vi "Check Histogram Options.vi"(8 "error in (no error)":errorcluster, 11 "Histogram Options in":T1 {"Max Histogram Size" format="%.0e"}) -> (0 "error out":errorcluster, 1 "Cancelled?":bool, 3 "Histogram Options out":T1 {"Max Histogram Size" format="%.0e"})   [LabVIEW 2021, in "Histogram Window.lvlib"]
uses:
  Histogram Window.lvlib
  Linear Histogram Options.ctl
  Histogram Bin Option.ctl
  Histogram Bin Position.ctl
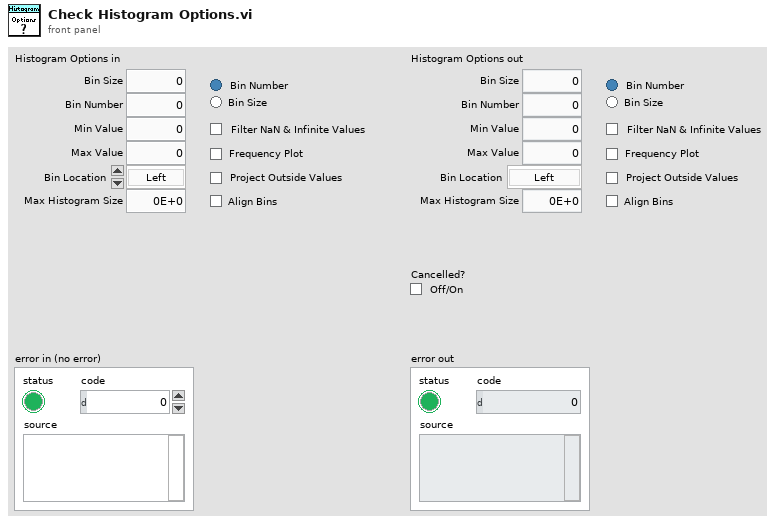
[diagram p1: front panel]
types:
  T1 = typedef "Histogram Window.lvlib/Linear Histogram Options.ctl" = cluster{"Bin Size":dbl, "Bin Number":i32, "Bin Option":T2, "Min Value":dbl, "Max Value":dbl, "Filter NaN & Infinite Values":bool, "Frequency Plot":bool, "Align Bins":bool, "Bin Location":T3, "Project Outside Values":bool, "Max Histogram Size":i32}
  T2 = typedef "Histogram Window.lvlib/Histogram Bin Option.ctl" = enum32{"Bin Number", "Bin Size"}
  T3 = typedef "Histogram Window.lvlib/Histogram Bin Position.ctl" = enum16{"Left", "Center", "Right"}
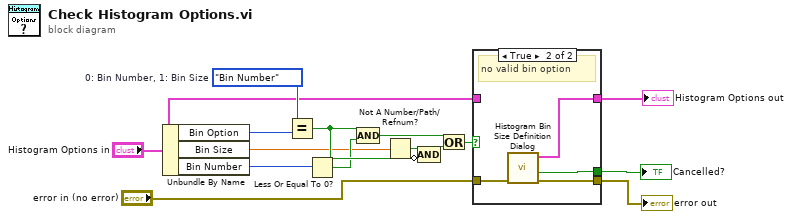
[diagram p0: block diagram]
diagram:
  w9 = Histogram_Bin_Option."Bin Number"  # 0: Bin Number, 1: Bin Size
  n1 = Unbundle By Name("Histogram Options in") -> ("Bin Option"=w8:T2, "Bin Size"=w5:dbl, "Bin Number"=w7:i32)
  n2 = Equal?(x=w9, y=w8) -> (x = y?=w12:bool)
  n3 = Less Or Equal To 0?(x=w7) -> (x <= 0?=w10:bool)
  n4 = Compound Arithmetic op=AND(w12, w10) -> (w13:bool)
  n5 = Not A Number/Path/Refnum?(number/path/refnum=w5) -> (NaN/Path/Refnum?=w11:bool)
  n6 = Compound Arithmetic op=AND(w11, invert w12) -> (w14:bool)
  n7 = Or(x=w13, y=w14) -> (x .or. y?=w15:bool)
  n8 = case shown="True" w15 {
    tunnel: [_ w19] -> w2
    tunnel: [w17 w21] -> w3
    tunnel: "error in (no error)" -> [w17 w20]
    tunnel: [w16 w18] -> w4
    tunnel: "Histogram Options in" -> [w16 _]
    frame False {
    }
    frame True {
      # "no valid bin option"
      n9 = call "Histogram Bin Size Definition Dialog.vi"("error in (no error)"=w20) -> ("error out"=w21:errorcluster, "Cancelled?"=w19:bool, "Histogram Options"=w18:T1)  [unwired: 8 in]
    }
  }
  "Histogram Options out" <- w4
  "error out" <- w3
  "Cancelled?" <- w2
